vi "Prompt for Step--Update State Data.vi"(8 "error in (no error)":errorcluster, 9 "Data":variant, 10 "Argument":string, 11 "Assertion Step in":refnum<class "Assertion Step.lvclass">) -> (0 "error out":errorcluster, 3 "Assertion Step out":refnum<class "Assertion Step.lvclass">)   [LabVIEW 2020, in "MacroAssert.lvlib" / "Assertion Step.lvclass"]
doc: "Updates the state data within the \"Prompt for Step\" VI."
uses:
  Assertion Step.lvclass
  Step/Step.lvclass
  Assertion Step.lvclass/Assertion Step.ctl
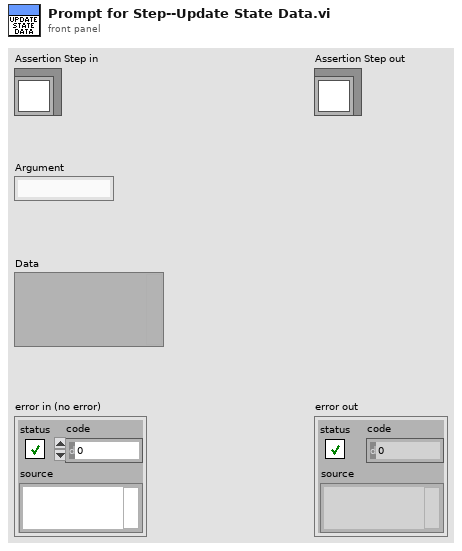
[diagram p1: front panel]
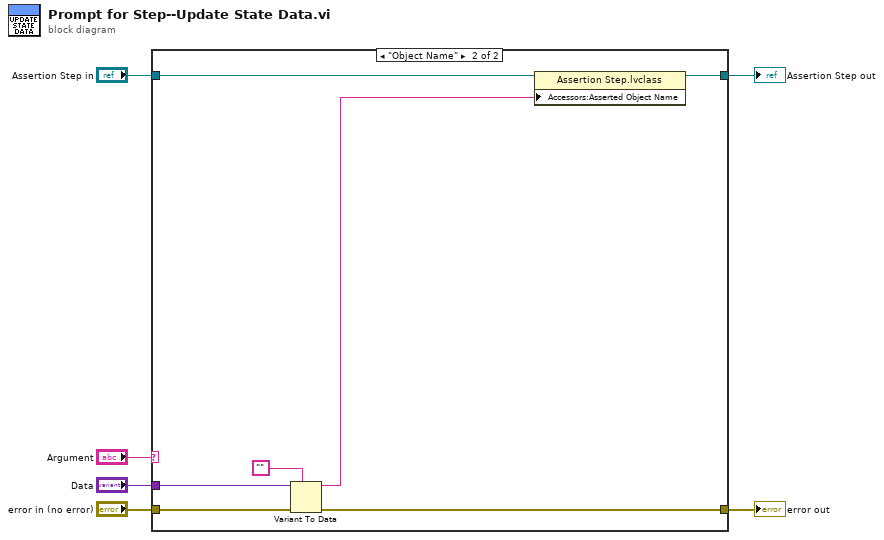
[diagram p0: block diagram]
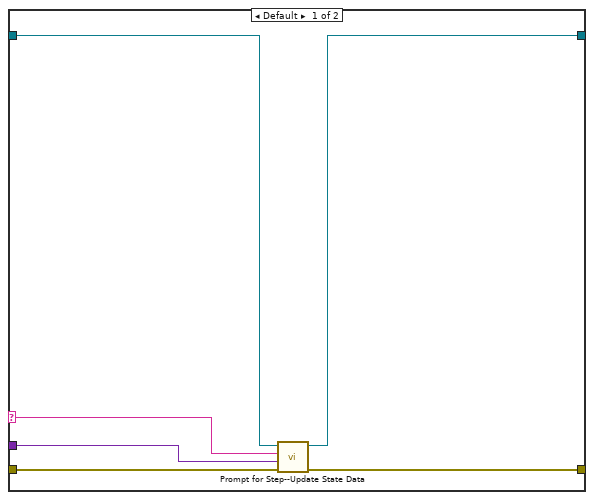
[diagram p2: hidden frame]
diagram:
  n1 = case shown="\"Object Name\"" "Argument" {
    selector: "Argument" -> [w9 _]
    tunnel: "Assertion Step in" -> [w8 w19]
    tunnel: "error in (no error)" -> [w12 w17]
    tunnel: [w7 w18] -> w1
    tunnel: [w11 w16] -> w5
    tunnel: "Data" -> [w10 w15]
    frame Default {
      n2 = call-parent "Prompt for Step--Update State Data.vi"("error in (no error)"=w12, "Data"=w10, "Argument"=w9, "Step in"=w8) -> ("error out"=w11:errorcluster, "Step out"=w7:refnum<class "Assertion Step.lvclass">)  [unwired: 6 in]
    }
    frame "Object Name" {
      n3 = Variant To Data(error in=w17, type="", Variant=w15) -> (data=w14:string, error out=w16:errorcluster)
      n4 = property class="Assertion Step.lvclass"(reference=w19, "Accessors:Asserted Object Name"=w14) -> (reference out=w18:refnum<class "Assertion Step.lvclass">)  [unwired: 1 in, 1 out]
    }
  }
  "error out" <- w5
  "Assertion Step out" <- w1
